vi "ForwardToTarget.vi"   [LabVIEW 2016, in "Project 2 LabVIEW.lvrbt"]
uses:
  Project 2 LabVIEW.lvrbt
  <vilib>/NXT/Block Support/NXT_OutputPort.ctl
  <vilib>/NXT/Dual Mode Library/Waits/Wait_Num.vi
  <vilib>/NXT/NXTIO Xnodes/NXTIONodeSubVIs/NXTMoveMotors.vi
  <vilib>/NXT/NXTIO Xnodes/NXTIONodeSubVIs/NXTStopMotors.vi
  <vilib>/NXT/NXTIO Xnodes/AddressXNode/NXTIOAddress.xnode
  <vilib>/NXT/NXTIO Xnodes/NXTIOXNode/NXTIO.xnode
  <vilib>/NXT/Subs/LVHSConnector.ctl
  <vilib>/NXT/LegoClasses/BrickReference/BrickReference.lvclass
types:
  T1 = typedef "LVHSConnector.ctl" = refnum<class "BrickReference.lvclass">
  T2 = typedef "NXT_OutputPort.ctl" = u8
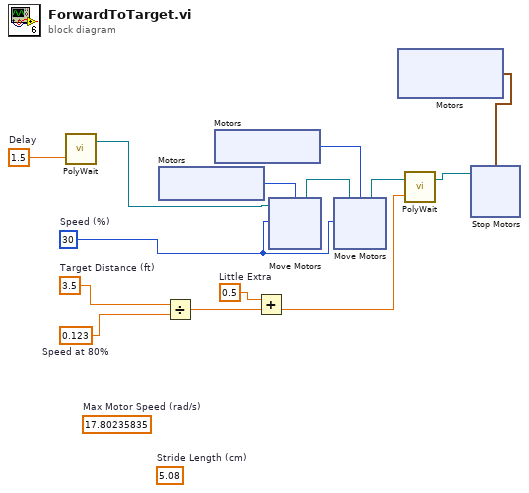
[diagram p0: block diagram]
diagram:
  w4 = 1.5  # Delay
  w5 = 0.5  # Little Extra
  w8 = 0.123  # Speed at 80%
  (unwired) 5.08  # Stride Length (cm)
  (unwired) 17.80235835  # Max Motor Speed (rad/s)
  w12 = 30  # Speed (%)
  w9 = 3.5  # Target Distance (ft)
  n1 = call-poly <vilib>:"PolyWait.vi"("Time (1 sec)"=w4) -> ("NXT/EV3"=w3:T1)  [unwired: 3 in]
  n2 = xnode "Motors"() -> ("Motor"=w13:T2)
  n3 = Divide(x=w9, y=w8) -> (x/y=w7:dbl)
  n4 = xnode "Motors"() -> ("Motor"=w14:T2)
  n5 = Add(x=w5, y=w7) -> (x+y=w6:dbl)
  n6 = xnode "Move Motors"("Power/Speed 1"=w12, "Motors"=w13, "NXT/EV3"=w3) -> ("NXT/EV3"=w11:T1)
  n7 = xnode "Move Motors"("Power/Speed 1"=w12, "Motors"=w14, "NXT/EV3"=w11) -> ("NXT/EV3"=w10:T1)
  n8 = xnode "Motors"() -> ("Motor"=w1:cluster{"Port":T2, "Port":T2})
  n9 = call-poly <vilib>:"PolyWait.vi"("Time (1 sec)"=w6, "NXT/EV3"=w10) -> ("NXT/EV3"=w2:T1)  [unwired: 2 in]
  n10 = xnode "Stop Motors"("Motors"=w1, "NXT/EV3"=w2) -> ()  [unwired: 1 out]
